vi "push to SQL with formeting to cluster.vi"(8 "error in (no error) 3":errorcluster, 10 "Table Name":string="Detailed_Report", 11 "array w/ subset deleted 2":string[][](array[string])) -> (0 "error Out (no error) 2":errorcluster)   [LabVIEW 2017]
uses:
  <vilib>/Utility/error.llb/whitespace.ctl
  SQL/SQL/SQL_DB-Enum.ctl
  Detailed Report/Controls/Detailed_Reports_Columns.ctl
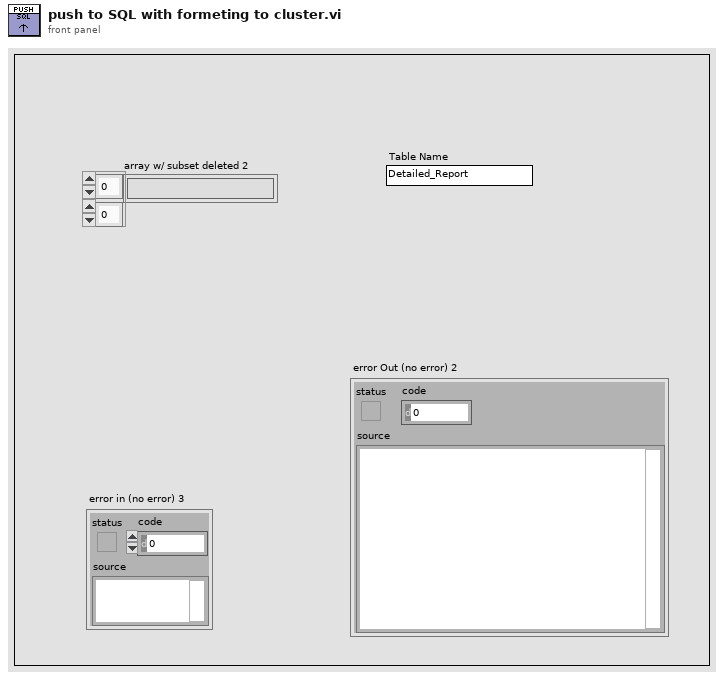
[diagram p1: front panel]
types:
  T1 = cluster{"barcode":string, "Time Stamp":string, "user name":string, "Shift":string, "Model":string, "Variant":string, "Testname":string, "test type":string, "Excepted Value":string, "hl":string, "ll":string, "obtained value":string, "result":string, "cycle time":string, "nip code":string}
  T2 = typedef "SQL_DB-Enum.ctl" = enum16{"INI DATA", "Open Connections", "Query", "Update Table", "Get Full Report", "Get Serial Numbers", "Get Table Columns", "Get Table Names", "Check & Create Table", "Close Connection"}
  T3 = typedef "Detailed_Reports_Columns.ctl" = string[]
  T4 = typedef "whitespace.ctl" = u16
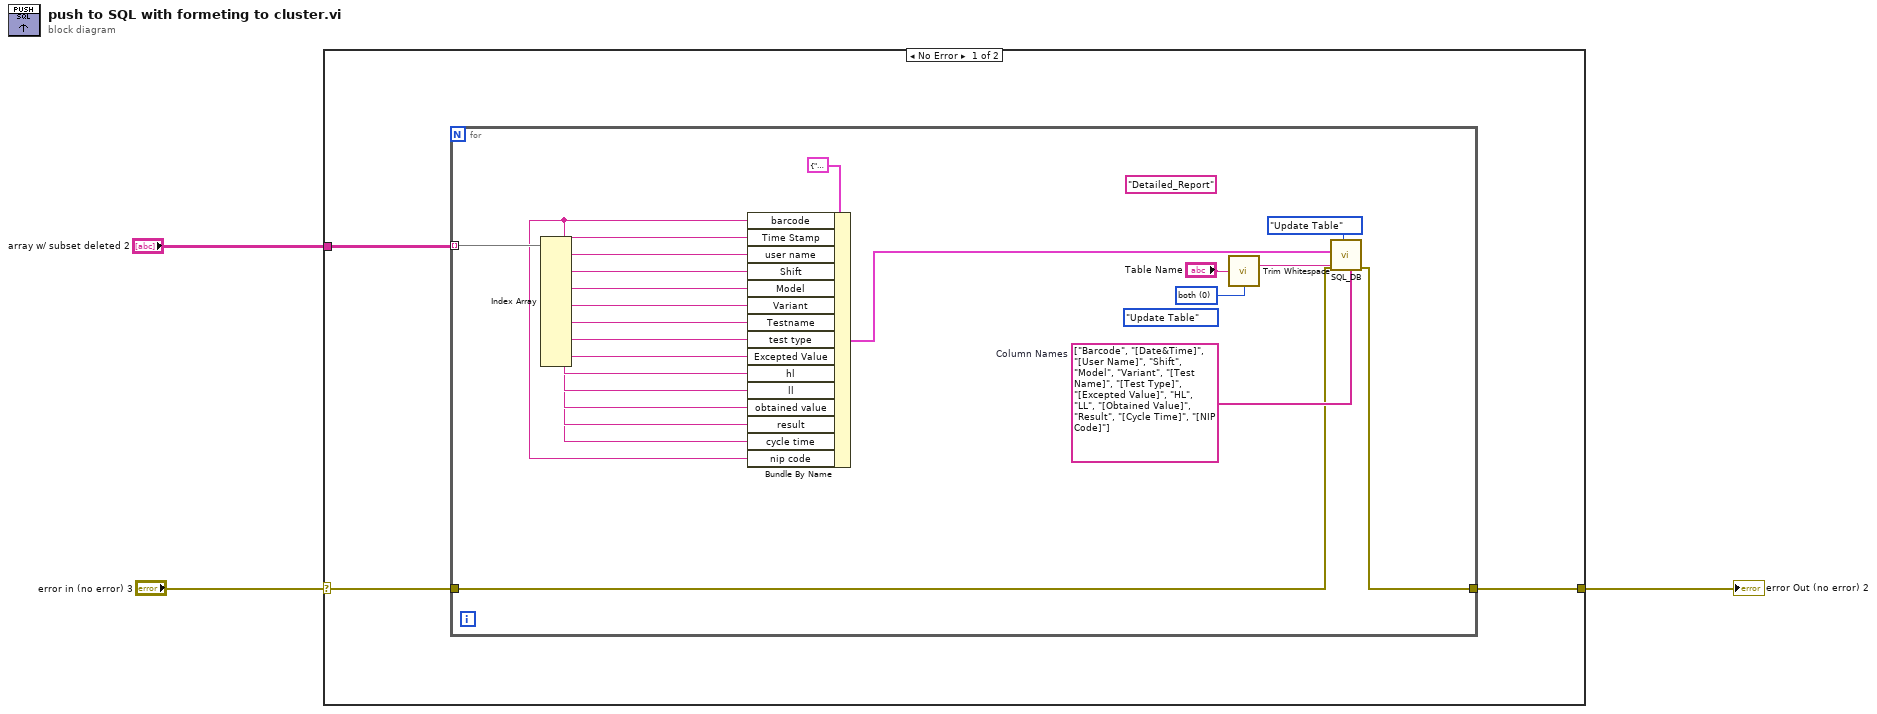
[diagram p0: block diagram]
diagram:
  n1 = case shown="No Error" "error in (no error) 3" {
    selector: "error in (no error) 3" -> [w4 w31]
    tunnel: "array w/ subset deleted 2" -> [w6 _]
    tunnel: [w5 w31] -> w2
    frame No Error {
      n2 = for {
        tunnel: w6 -> [w28] mode=indexing
        tunnel: [w9] -> w5
        tunnel: w4 -> [w8]
        (unwired) "Detailed_Report" ("Table Name")
        w10 = T3 ["Barcode", "[Date&Time]", "[User Name]", "Shift", "Model", "Variant", "[Test Name]", "[Test Type]", "[Excepted Value]", "HL", "LL", "[Obtained Value]", "Result", "[Cycle Time]", "[NIP Code]"]  # Column Names
        (unwired) SQL_DB-Enum."Update Table" ("CTRL")
        w12 = T4 0 items=["both", "start of string", "end of string"] ("location (both)")
        n3 = Index Array(array=w28) -> (element #1=w13:string, element #2=w26:string, element #3=w25:string, element #4=w24:string, element #5=w23:string, element #6=w22:string, element #7=w21:string, element #8=w20:string, element #9=w19:string, element #10=w18:string, element #11=w17:string, element #12=w16:string, element #13=w15:string, element #14=w14:string)  [unwired: 14 in]
        n4 = Bundle By Name(cluster=T1 {"barcode"="barcode", "Time Stamp"="2019-12-13 20:24:09.05", "user name"="1", "Shift"="shifr", "Model"="model", "Variant"="variant", "Testname"="test name", "test type"="test type", "Excepted Value"="test type", "hl"="hl", "ll"="ll", "obtained value"="obtained", "result"="resrut", "cycle time"="Cycle time", "nip code"="nip code"}, "barcode"=w13, "Time Stamp"=w26, "user name"=w25, "Shift"=w24, "Model"=w23, "Variant"=w22, "Testname"=w21, "test type"=w20, "Excepted Value"=w19, "hl"=w18, "ll"=w17, "obtained value"=w16, "result"=w15, "cycle time"=w14, "nip code"=w13) -> (w29:T1)
        n5 = call <vilib>:"Trim Whitespace.vi"("string"="Table Name", "location (both)"=w12) -> ("trimmed string"=w11:string)
        n6 = call "SQL_DB.vi"("Column Names"=w10, "Table Name"=w11, "CTRL"=SQL_DB-Enum."Update Table", "error in (no error)"=w8, "data to Update"=w29) -> ("error in (no error) 2"=w9:errorcluster)  [unwired: 4 in, 2 out]
      }
    }
    frame Error {
    }
  }
  "error Out (no error) 2" <- w2
